vi "InconListToOpenList.vi"(11 "RVCLibrary_Bug2 in":refnum<class "RVCLibrary_Bug2.lvclass">) -> (3 "RVCLibrary_Bug2 out":refnum<class "RVCLibrary_Bug2.lvclass">)   [LabVIEW 2013, in "RVCLibrary_Bug2.lvclass"]
uses:
  RVCLibrary_Bug2.lvclass
  RVCLibrary_Bug2.lvclass/RVCLibrary_Bug2.ctl
  <vilib>/robotics/Navigation/shared/InconsistentList/NI_Robotics_InconsistentList.lvclass
  <vilib>/robotics/Navigation/shared/MapNode/AbstractDstarNode/NI_Robotics_AbstractDstarNode.lvclass
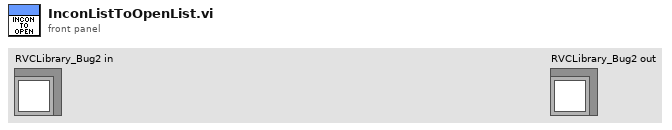
[diagram p1: front panel]
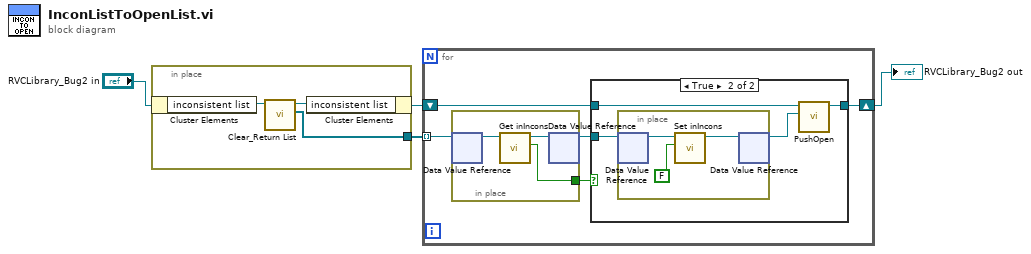
[diagram p0: block diagram]
diagram:
  n1 = in-place {
    in-place-border: [w5] -> w3
    n2 = in-place-cluster #1("RVCLibrary_Bug2 in") -> ("inconsistent list"=w7:refnum<class "NI_Robotics_InconsistentList.lvclass">)
    n3 = call <vilib>:"Clear_Return List.vi"("InconsistentList in"=w7) -> ("nodes"=w5:refnum<data-value>[], "InconsistentList out"=w6:refnum<class "NI_Robotics_InconsistentList.lvclass">)  [unwired: 8 in, 1 out]
    n4 = in-place-cluster #1("inconsistent list"=w6) -> (w4:refnum<class "RVCLibrary_Bug2.lvclass">)
  }
  n5 = for {
    shift-right: [w11] -> w1
    shift-left: w4 -> [w12]
    tunnel: w3 -> [w10] mode=indexing
    n6 = in-place {
      in-place-border: [w21] -> w8
      n7 = in-place-dvr #2(w10) -> (w23:refnum<class "NI_Robotics_AbstractDstarNode.lvclass">)  [unwired: 1 out]
      n8 = call <vilib>:"Get inIncons.vi"("AbstractDstarNode in"=w23) -> ("inIncons"=w21:bool, "AbstractDstarNode out"=w22:refnum<class "NI_Robotics_AbstractDstarNode.lvclass">)  [unwired: 9 in]
      n9 = in-place-dvr #2(w22) -> (w9:refnum<data-value>)  [unwired: 1 out]
    }
    n10 = case shown="True" w8 {
      tunnel: w12 -> [w13 w17]
      tunnel: [w13 w16] -> w11
      tunnel: w9 -> [_ w15]
      frame False {
      }
      frame True {
        n11 = in-place {
          n12 = in-place-dvr #3(w15) -> (w20:refnum<class "NI_Robotics_AbstractDstarNode.lvclass">)  [unwired: 1 out]
          n13 = call <vilib>:"Set inIncons.vi"("inIncons"=FALSE, "AbstractDstarNode in"=w20) -> ("AbstractDstarNode out"=w19:refnum<class "NI_Robotics_AbstractDstarNode.lvclass">)  [unwired: 9 in]
          n14 = in-place-dvr #3(w19) -> (w14:refnum<data-value>)  [unwired: 1 out]
        }
        n15 = call "PushOpen.vi"("node ref in"=w14, "RVCLibrary_Bug in"=w17) -> ("RVCLibrary_Bug out"=w16:refnum<class "RVCLibrary_Bug2.lvclass">)  [unwired: 8 in, 1 out]
      }
    }
  }
  "RVCLibrary_Bug2 out" <- w1
